vi "Write.vi"(8 "error in (no error)":errorcluster, 10 "Array":string[][](array[string]), 11 "TXT in":refnum<class "TXT.lvclass">) -> (0 "error out":errorcluster, 3 "TXT out":refnum<class "TXT.lvclass">)   [LabVIEW 2014, in "TXT.lvclass"]
uses:
  TXT.lvclass
  TXT.lvclass/TXT.ctl
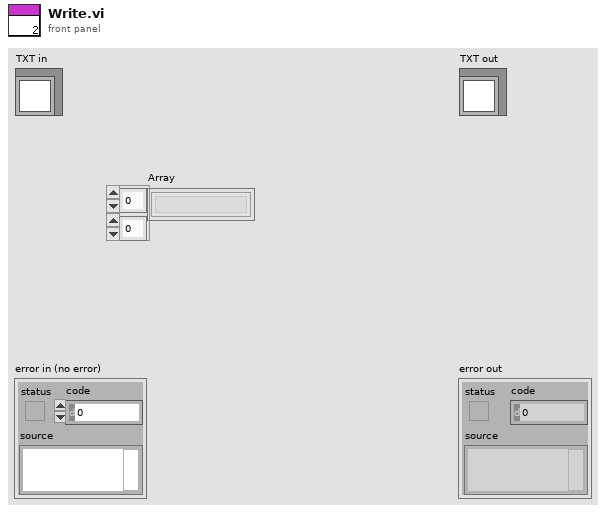
[diagram p1: front panel]
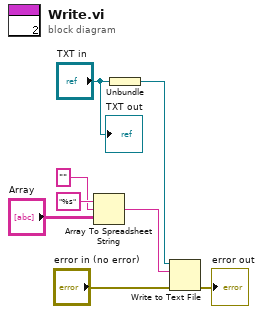
[diagram p0: block diagram]
diagram:
  n1 = Array To Spreadsheet String(delimiter (Tab)="", array="Array", 3:"%s") -> (spreadsheet string=w3:string)
  n2 = Unbundle("TXT in") -> (w6:refnum<file>)
  n3 = Write to Text File(file (use dialog)=w6, text=w3, error in="error in (no error)") -> (error out=→"error out":errorcluster)  [unwired: 1 in, 2 out]
  "TXT out" <- "TXT in"
